vi "23384_Davis_Poku_Amankwa_Amankwa.DavisPoku.MNE1201.7.7a_348263_563713699.vi"() -> ()   [LabVIEW 2018]
panel:
  in  "?":bool
  out "Output":dbl
  in  "Input":dbl
  in  "Conversion Mode":enum16{"Cto F", "F to C"}(ring)=enum."F to C"
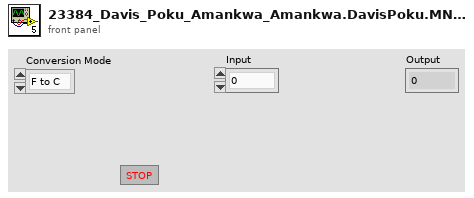
[diagram p1: front panel]
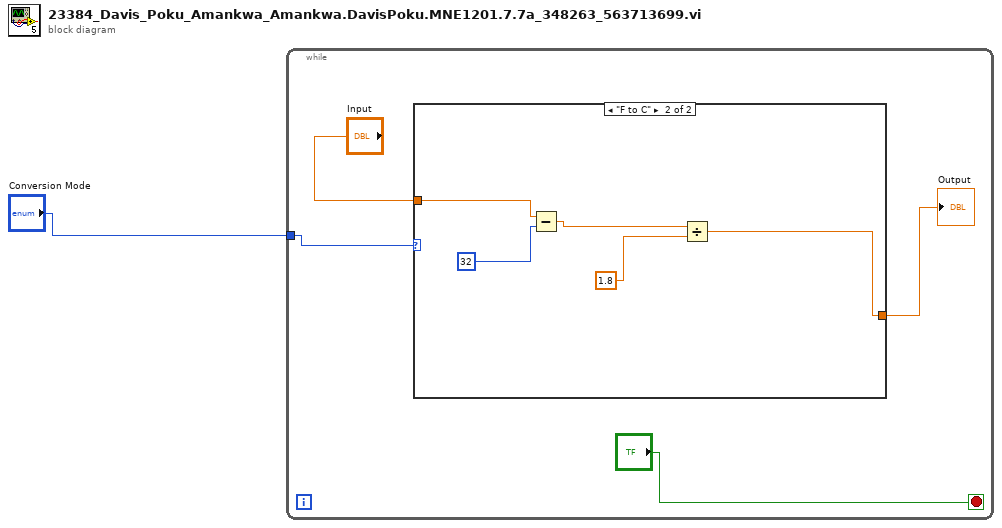
[diagram p0: block diagram]
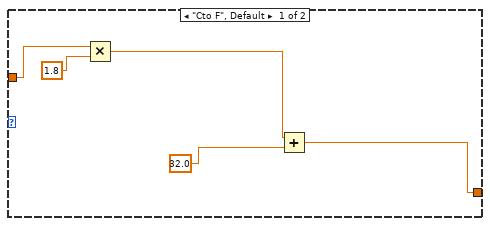
[diagram p2: hidden frame]
diagram:
  n1 = while {
    tunnel: "Conversion Mode" -> [w5]
    stop <- "?" stop-if-true
    n2 = case shown="\"F to C\"" w5 {
      tunnel: [w10 w11] -> w4
      tunnel: "Input" -> [w9 w14]
      frame "Cto F", Default {
        n3 = Multiply(x=w9, y=1.8) -> (x*y=w7:dbl)
        n4 = Add(x=w7, y=32.0) -> (x+y=w10:dbl)
      }
      frame "F to C" {
        n5 = Subtract(x=w14, y=32) -> (x-y=w13:dbl)
        n6 = Divide(x=w13, y=1.8) -> (x/y=w11:dbl)
      }
    }
    "Output" <- w4
  }
